vi "wielomiany_rts1.vi"() -> ()   [LabVIEW 2019]
panel:
  out "y:":string
  in  "c":dbl
  in  "b":dbl
  in  "a":dbl
  in  "X":dbl
  in  "Enum":T1(ring)
  in  "?":bool
  in  "?":bool
  # "y = a+bx+ cx^2"
  # "y = a+bx^2 - 3x^4"
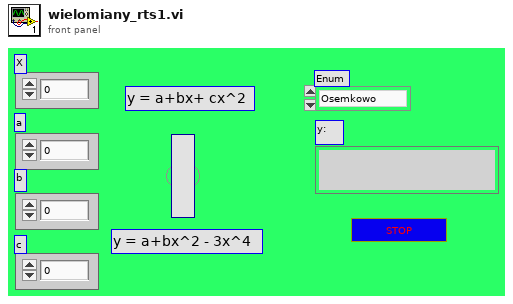
[diagram p1: front panel]
types:
  T1 = enum16{"Osemkowo", "Dziesietnie", "Szesnastkowo"}
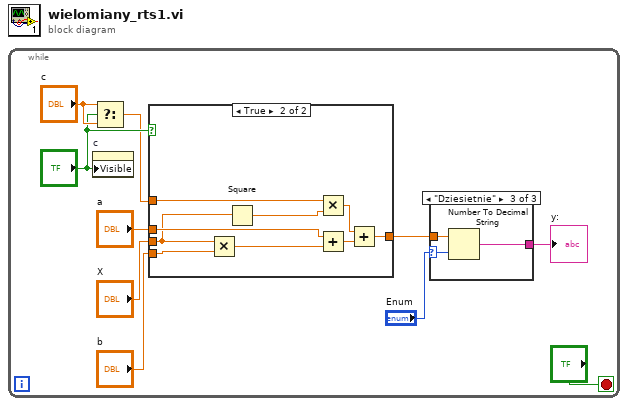
[diagram p0: block diagram]
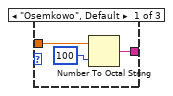
[diagram p2: hidden frame]
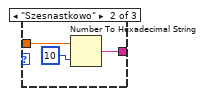
[diagram p3: hidden frame]
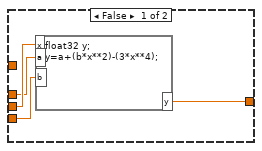
[diagram p4: hidden frame]
diagram:
  n1 = while {
    stop <- "?" stop-if-true
    n2 = property on="c" class="DigNum (strict)"("Visible"="?") -> ()  [unwired: 2 in, 2 out]
    n3 = Select(t="c", s="?", f="c") -> (s? t:f=w4:dbl)
    n4 = case shown="True" "?" {
      tunnel: "X" -> [w23 w28]
      tunnel: "a" -> [w22 w31]
      tunnel: "b" -> [w21 w32]
      tunnel: [w20 w24] -> w2
      tunnel: w4 -> [_ w29]
      frame False {
        n5 = formula code="float32 y;\ny=a+(b*x**2)-(3*x**4);"("x"=w23, "a"=w22, "b"=w21) -> ("y"=w20:sgl)
      }
      frame True {
        n6 = Multiply(x=w28, y=w32) -> (x*y=w30:dbl)
        n7 = Square(x=w28) -> (x^2=w27:dbl)
        n8 = Multiply(x=w29, y=w27) -> (x*y=w26:dbl)
        n9 = Add(x=w31, y=w30) -> (x+y=w25:dbl)
        n10 = Add(x=w26, y=w25) -> (x+y=w24:dbl)
      }
    }
    n11 = case shown="\"Dziesietnie\"" "Enum" {
      selector: "Enum" -> [_ _ w18]
      tunnel: w2 -> [w13 w16 w19]
      tunnel: [w11 w14 w17] -> w1
      frame "Osemkowo", Default {
        n12 = Number To Octal String(1:i16 100 ("width (-)"), 2:w13) -> (0:w11:string)
      }
      frame "Szesnastkowo" {
        n13 = Number To Hexadecimal String(1:i16 10 ("width (-)"), 2:w16) -> (0:w14:string)
      }
      frame "Dziesietnie" {
        n14 = Number To Decimal String(number=w19, width (-)=w18) -> (decimal integer string=w17:string)
      }
    }
    "y:" <- w1
  }
